vi "ConvertGoop3ToGoop4_UpdateNewVICallers.vi"(8 "error in (no error)":errorcluster, 10 "InsertAlwaysCopy":bool, 11 "ViRef":refnum<vi>) -> (0 "error out":errorcluster, 3 "ViRefOut":refnum<vi>)   [LabVIEW 2020]
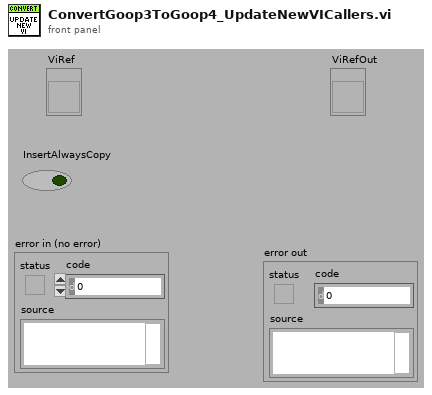
[diagram p1: front panel]
types:
  T1 = enum16{"Create or look up existing", "Look up existing"}
  T2 = enum16{"Create", "Create or look up existing", "Look up existing"}
  T3 = enum32{"invalid lock state", "Not Locked", "Locked (No Password)", "Password-protected"}
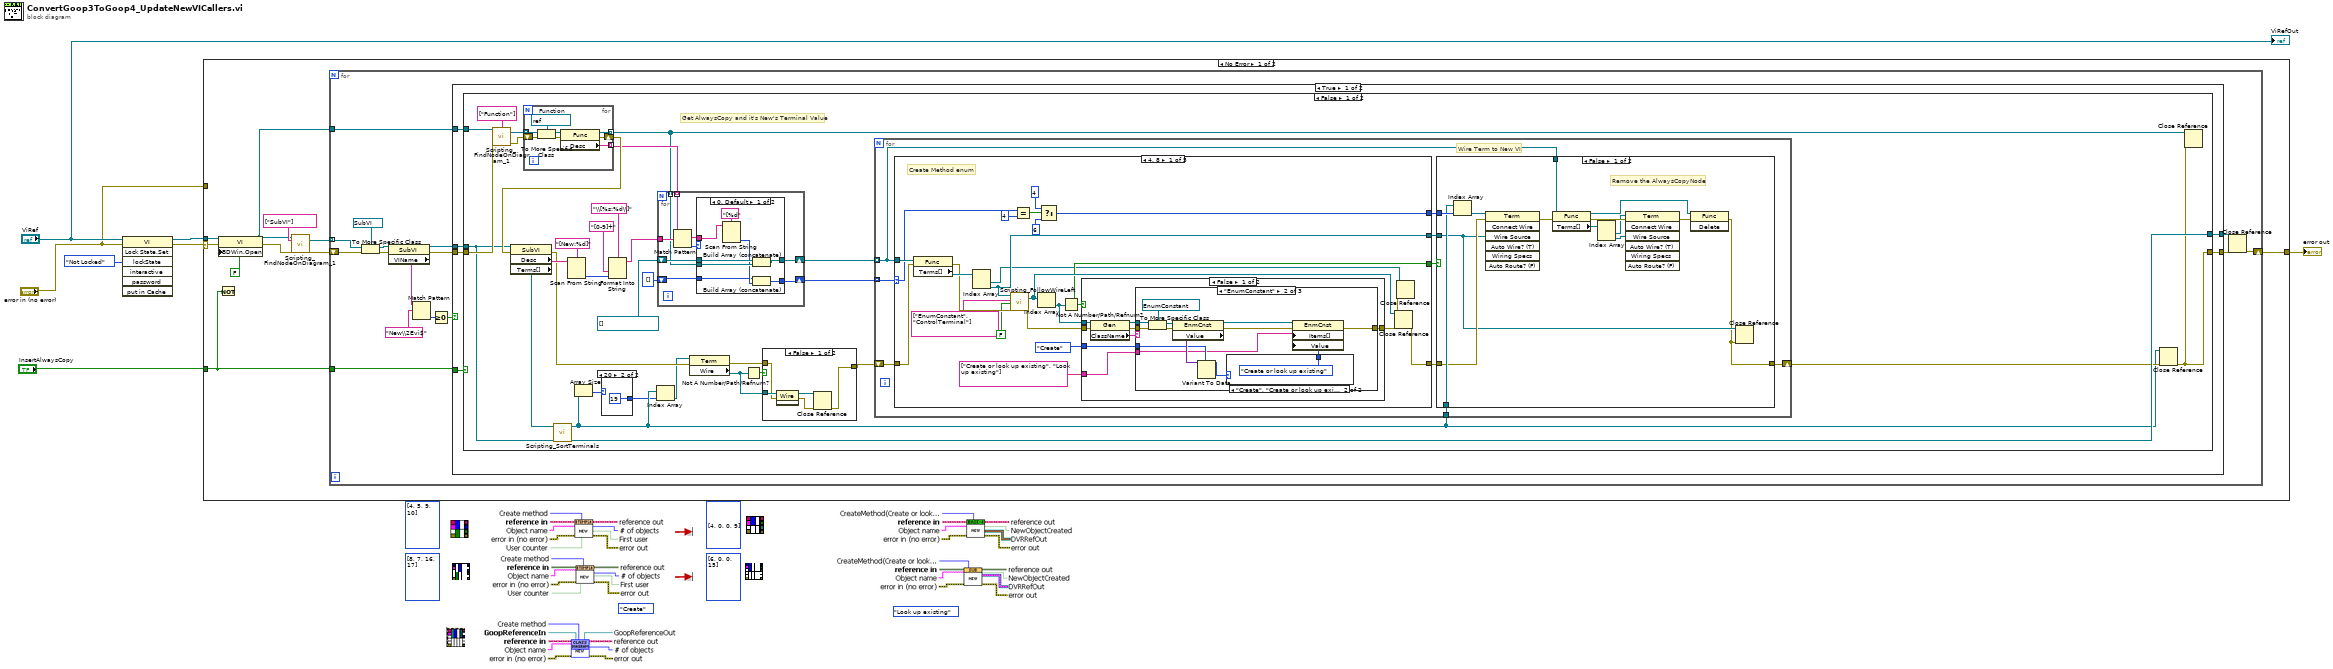
[diagram p0: block diagram]
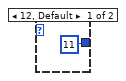
[diagram p3: hidden frame]
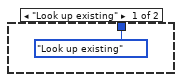
[diagram p6: hidden frame]
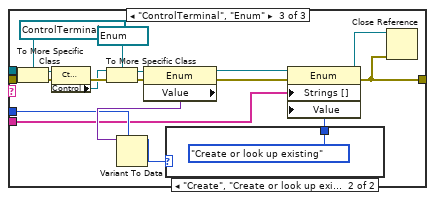
[diagram p7: hidden frame]
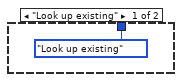
[diagram p8: hidden frame]
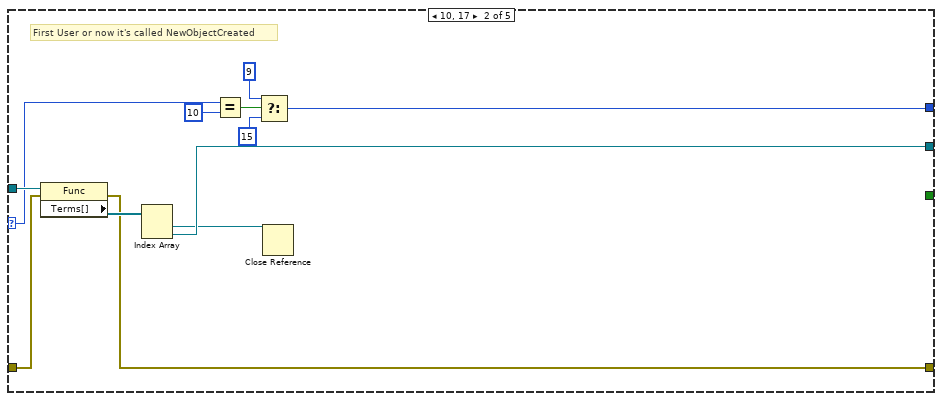
[diagram p10: hidden frame]
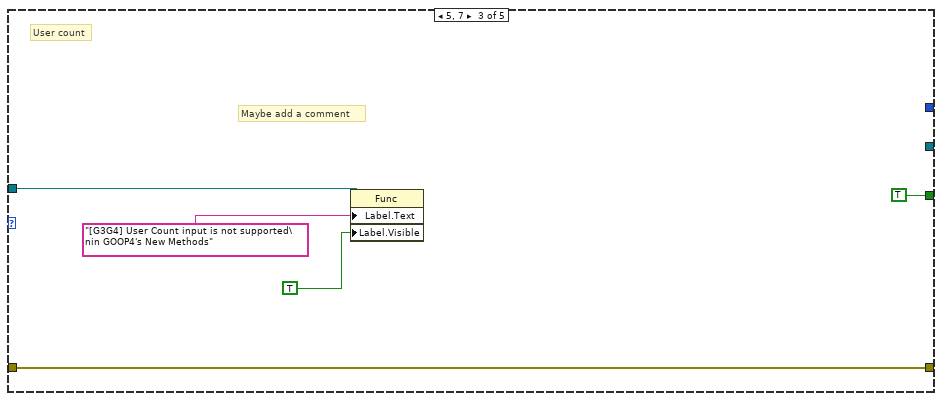
[diagram p11: hidden frame]
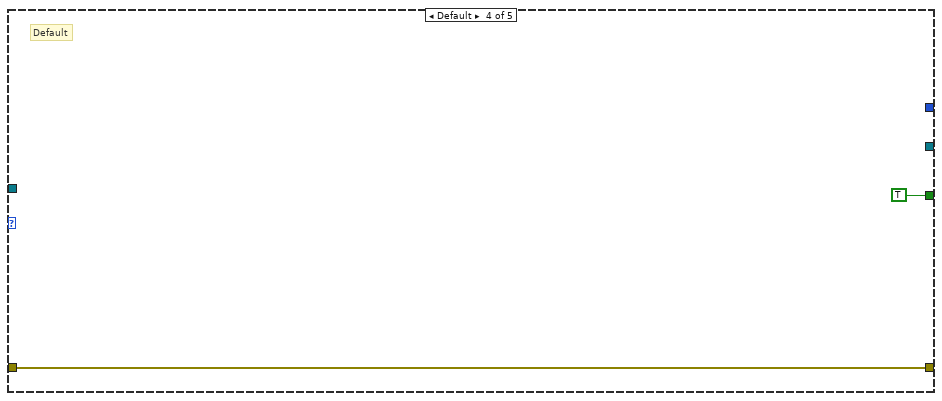
[diagram p12: hidden frame]
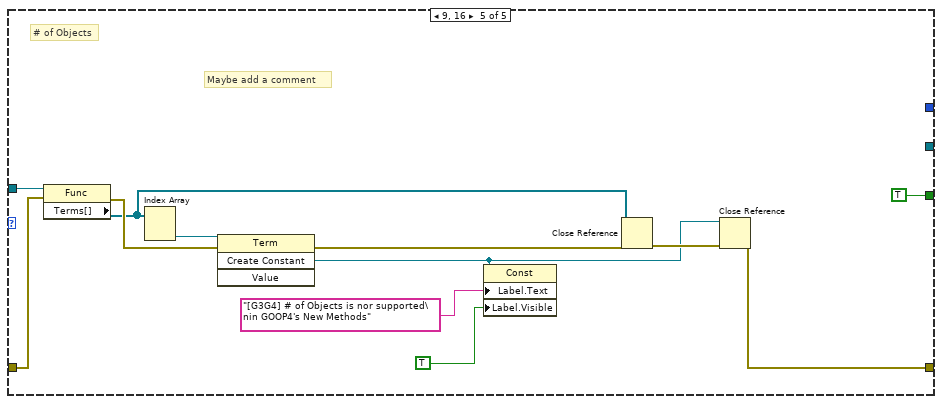
[diagram p13: hidden frame]
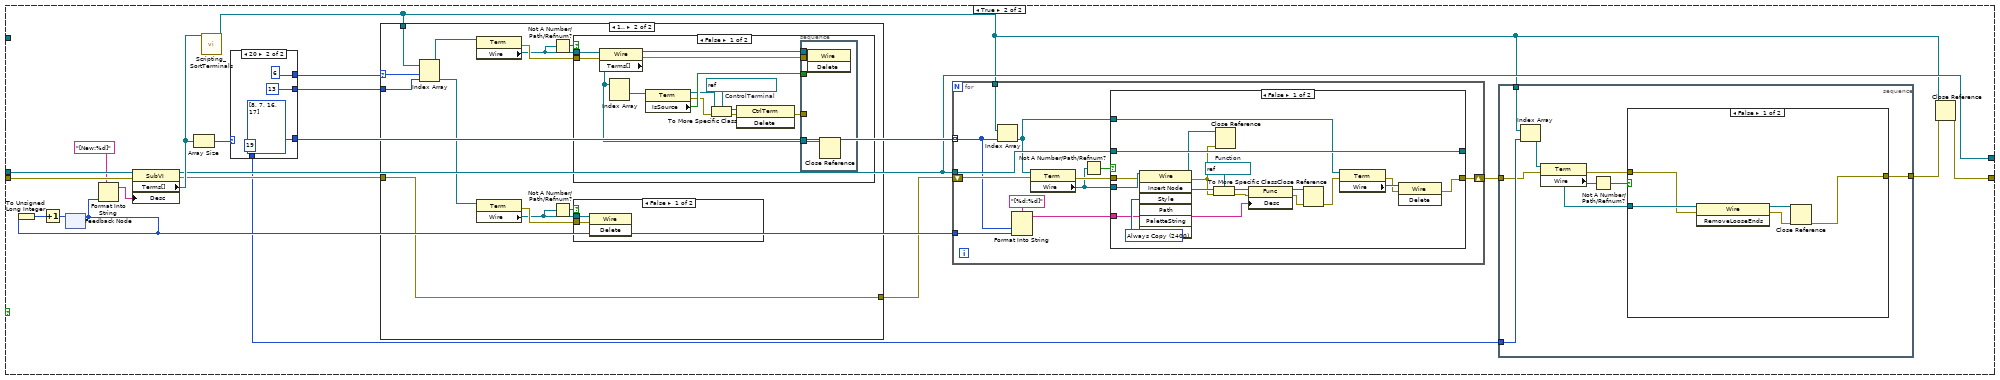
[diagram p15: hidden frame]
diagram:
  (unwired) i32[] [4, 0, 0, 9]
  (unwired) i32[] [6, 0, 0, 15]
  (unwired) T1."Look up existing" ("CreateMethod(Create or look up existing)")
  (unwired) T2."Create" ("Create method")
  (unwired) i32[] [4, 5, 9, 10]
  (unwired) i32[] [8, 7, 16, 17]
  n1 = invoke class="VI" method="Lock State.Set"(reference="ViRef", error in="error in (no error)", "lockState"=T3."Not Locked" ("Lock State")) -> (reference out=w5:refnum<vi>, error out=w2:errorcluster)  [unwired: 4 in, 5 out]
  n2 = case shown="No Error" w2 {
    selector: w2 -> [w11 _]
    tunnel: [w14 w334] -> w7
    tunnel: w5 -> [w12 _]
    tunnel: "error in (no error)" -> [_ w334]
    tunnel: "InsertAlwaysCopy" -> [w9 _]
    frame No Error {
      n3 = property class="VI"(reference=w12, error in=w11, "BDWin.Open"=FALSE ("Block Diagram Window:Open")) -> (reference out=w10:refnum<vi>, error out=w13:errorcluster)
      n4 = Not(x=w9) -> ()  [unwired: 1 out]
      n5 = call <resource>:"Scripting_FindNodeOnDiagram_1.vi"("ViRef(Ignored If Not Wired)"=w10, "NodeTypesToSearchFor"=string[] ["SubVI"], "error in (no error)"=w13) -> ("Nodes"=w16:refnum<vi>[], "error out"=w15:errorcluster)  [unwired: 15 in]
      n6 = for {
        tunnel: w16 -> [w33] mode=indexing
        shift-right: [w25] -> w14
        shift-left: w15 -> [w31]
        tunnel: w9 -> [w19]
        tunnel: w10 -> [w18]
        n7 = To More Specific Class(target class=refnum<vi> refnum ("WhileLoop"), reference=w33, error in=w31) -> (specific class reference=w30:refnum<vi>, error out=w29:errorcluster)
        n8 = property class="SubVI"(reference=w30, error in=w29) -> (reference out=w28:refnum<vi>, error out=w27:errorcluster, "VIName"=w20:string)
        n9 = Match Pattern(string=w20, regular expression="New\\2Evi$") -> (offset past match=w22:i32)  [unwired: 1 in, 3 out]
        n10 = Greater Or Equal To 0?(x=w22) -> (x >= 0?=w23:bool)
        n11 = case shown="True" w23 {
          tunnel: w28 -> [w39 w332]
          tunnel: w27 -> [w38 w333]
          tunnel: [w37 w333] -> w26
          tunnel: [w34 w332] -> w24
          tunnel: w19 -> [w36 _]
          tunnel: w18 -> [w35 _]
          frame True {
            n12 = case shown="False" w36 {
              tunnel: w39 -> [w53 w248]
              tunnel: w38 -> [w69 w245]
              tunnel: [w49 w242] -> w37
              tunnel: w35 -> [w68 _]
              tunnel: [w53 w237] -> w34
              frame False {
                # "Get AlwaysCopy and it's New's Terminal Value"
                n13 = call <resource>:"Scripting_FindNodeOnDiagram_1.vi"("ViRef(Ignored If Not Wired)"=w68, "NodeTypesToSearchFor"=string[] ["Function"], "error in (no error)"=w69) -> ("Nodes"=w67:refnum<vi>[], "error out"=w66:errorcluster)  [unwired: 15 in]
                n14 = for {
                  tunnel: w67 -> [w226] mode=indexing
                  tunnel: [w225] -> w60 mode=indexing
                  tunnel: [w224] -> w50 mode=indexing
                  shift-right: [w222] -> w65
                  shift-left: w66 -> [w223]
                  w227 = refnum<vi> refnum  # Function
                  n15 = To More Specific Class(target class=w227, reference=w226, error in=w223) -> (specific class reference=w228:refnum<vi>, error out=w221:errorcluster)
                  n16 = property class="Func"(reference=w228, error in=w221) -> (reference out=w224:refnum<vi>, error out=w222:errorcluster, "Desc"=w225:string)
                }
                n17 = property class="SubVI"(reference=w53, error in=w65) -> (error out=w45:errorcluster, "Desc"=w64:string, "Terms[]"=w52:refnum<vi>[])  [unwired: 1 out]
                n18 = call <resource>:"Scripting_SortTerminals.vi"("Terminals[]"=w52) -> ("TerminalsOut[]"=w47:refnum<vi>[])  [unwired: 8 in, 2 out]
                n19 = Scan From String(format string="[New:%d]", input string=w64) -> (output 1=w61:i32)  [unwired: 3 in, 3 out]
                n20 = Array Size(array=w47) -> (size(s)=w48:i32)
                n21 = case shown="20" w48 {
                  tunnel: [11 ("index") 19 ("index")] -> w46
                  frame 12, Default {
                  }
                  frame 20 {
                  }
                }
                n22 = Format Into String(format string="\\[%s:%d\\]", "[0-9]+" ("format string"), w61) -> (resulting string=w58:string)  [unwired: 2 in, 1 out]
                n23 = Index Array(array=w47, index=w46) -> (element=w44:refnum<vi>)
                n24 = for {
                  tunnel: w60 -> [w210] mode=indexing
                  tunnel: w58 -> [w209]
                  shift-right: [w206] -> w55
                  shift-left: refnum<vi>[] [] -> [w207]
                  tunnel: w50 -> [w205] mode=indexing
                  shift-right: [w204] -> w54
                  shift-left: i32[] [] -> [w203]
                  n25 = Match Pattern(string=w210, regular expression=w209) -> (match substring=w202:string, offset past match=w208:i32)  [unwired: 1 in, 2 out]
                  n26 = case shown="0, Default" w208 {
                    tunnel: w207 -> [w218 w220]
                    tunnel: [w217 w220] -> w206
                    tunnel: w205 -> [w216 _]
                    tunnel: w202 -> [w215 _]
                    tunnel: [w212 w219] -> w204
                    tunnel: w203 -> [w211 w219]
                    frame 0, Default {
                      n27 = Scan From String(format string="[%d", input string=w215) -> (output 1=w213:i32)  [unwired: 3 in, 3 out]
                      n28 = Build Array (concatenate)(w218, w216) -> (w217:refnum<vi>[])
                      n29 = Build Array (concatenate)(w211, w213) -> (w212:i32[])
                    }
                    frame -1 {
                    }
                  }
                }
                n30 = property class="Term"(reference=w44, error in=w45) -> (error out=w42:errorcluster, "Wire"=w40:refnum<vi>)  [unwired: 1 out]
                n31 = Not A Number/Path/Refnum?(number/path/refnum=w40) -> (NaN/Path/Refnum?=w43:bool)
                n32 = case shown="False" w43 {
                  tunnel: w40 -> [w75 _]
                  tunnel: w42 -> [w74 w76]
                  tunnel: [w71 w76] -> w41
                  frame False {
                    n33 = invoke class="Wire" method="RemoveLooseEnds"(reference=w75, error in=w74) -> (reference out=w73:refnum<vi>, error out=w72:errorcluster)  [unwired: 1 in, 1 out]
                    n34 = Close Reference(reference=w73, error in (no error)=w72) -> (error out=w71:errorcluster)
                  }
                  frame True {
                  }
                }
                n35 = for {
                  tunnel: w55 -> [w80] mode=indexing
                  tunnel: w54 -> [w87] mode=indexing
                  shift-right: [w79] -> w51
                  shift-left: w41 -> [w86]
                  tunnel: w47 -> [w83]
                  # "Wire Term to New VI"
                  n36 = case shown="4, 8" w87 {
                    selector: w87 -> [w114 w179 _ _ _]
                    tunnel: w80 -> [w124 w182 w184 _ w200]
                    tunnel: w86 -> [w123 w181 w187 w189 w193]
                    tunnel: [w109 w174 _ _ _] -> w84
                    tunnel: [w108 w172 w187 w189 w194] -> w85
                    tunnel: [w107 _ TRUE TRUE TRUE] -> w81
                    tunnel: [w106 w173 _ _ _] -> w82
                    frame 4, 8 {
                      # "Create Method enum"
                      n37 = property class="Func"(reference=w124, error in=w123) -> (error out=w121:errorcluster, "Terms[]"=w122:refnum<vi>[])  [unwired: 1 out]
                      n38 = Index Array(array=w122) -> (element #1=w103:refnum<vi>, element #2=w106:refnum<vi>)  [unwired: 2 in]
                      n39 = call <resource>:"Scripting_FollowWireLeft.vi"("Term Refnum"=w106, "NodeTypesToFind"=string[] ["EnumConstant", "ControlTerminal"], "CreateParentTerminals(False)"=FALSE, "error in"=w121) -> ("Nodes"=w115:refnum<vi>[], "error out"=w117:errorcluster)  [unwired: 12 in, 2 out]
                      n40 = Equal?(x=w114, y=4) -> (x = y?=w112:bool)
                      n41 = Index Array(array=w115) -> (element=w118:refnum<vi>)  [unwired: 1 in]
                      n42 = Select(t=4 ("y"), s=w112, f=6) -> (s? t:f=w109:i32)
                      n43 = Not A Number/Path/Refnum?(number/path/refnum=w118) -> (NaN/Path/Refnum?=w107:bool)
                      n44 = case shown="False" w107 {
                        tunnel: w118 -> [w132 _]
                        tunnel: w117 -> [w131 w170]
                        tunnel: T2."Create" ("Create method") -> [w127 _]
                        tunnel: [w126 w170] -> w104
                        tunnel: string[] ["Create or look up existing", "Look up existing"] ("Items[]") -> [w125 _]
                        frame False {
                          n45 = property class="Gen"(reference=w132, error in=w131) -> (reference out=w129:refnum<vi>, error out=w128:errorcluster, "ClassName"=w130:string)
                          n46 = case shown="\"EnumConstant\"" w130 {
                            tunnel: w129 -> [_ w146 w167]
                            tunnel: w128 -> [w133 w145 w166]
                            tunnel: w127 -> [_ w138 w162]
                            tunnel: [w133 w135 w150] -> w126
                            tunnel: w125 -> [_ w134 w158]
                            frame Default {
                            }
                            frame "EnumConstant" {
                              n47 = To More Specific Class(target class=refnum<vi> refnum ("reference"), reference=w146, error in=w145) -> (specific class reference=w143:refnum<vi>, error out=w142:errorcluster)
                              n48 = property class="EnmCnst"(reference=w143, error in=w142) -> (reference out=w141:refnum<vi>, error out=w140:errorcluster, "Value"=w139:variant)
                              n49 = Variant To Data(type=w138, Variant=w139) -> (data=w137:T2)  [unwired: 1 in, 1 out]
                              n50 = case shown="\"Create\", \"Create or look up existing\", Default" w137 {
                                tunnel: [T1."Look up existing" ("CreateMethod(Create or look up existing)") T1."Create or look up existing" ("CreateMethod(Create or look up existing)")] -> w136
                                frame "Look up existing" {
                                }
                                frame "Create", "Create or look up existing", Default {
                                }
                              }
                              n51 = property class="EnmCnst"(reference=w141, error in=w140, "Items[]"=w134, "Value"=w136) -> (error out=w135:errorcluster)  [unwired: 1 out]
                            }
                            frame "ControlTerminal", "Enum" {
                              n52 = To More Specific Class(target class=refnum<vi> refnum ("reference"), reference=w167, error in=w166) -> (specific class reference=w156:refnum<vi>, error out=w155:errorcluster)
                              n53 = property class="CtrlTerm"(reference=w156, error in=w155) -> (error out=w154:errorcluster, "Control"=w151:refnum<vi>)  [unwired: 1 out]
                              n54 = To More Specific Class(target class=refnum<vi> refnum ("reference"), reference=w151, error in=w154) -> (specific class reference=w152:refnum<vi>, error out=w153:errorcluster)
                              n55 = property class="Enum"(reference=w152, error in=w153) -> (reference out=w165:refnum<vi>, error out=w164:errorcluster, "Value"=w163:variant)
                              n56 = Variant To Data(type=w162, Variant=w163) -> (data=w161:T2)  [unwired: 1 in, 1 out]
                              n57 = case shown="\"Create\", \"Create or look up existing\", Default" w161 {
                                tunnel: [T1."Look up existing" ("CreateMethod(Create or look up existing)") T1."Create or look up existing" ("CreateMethod(Create or look up existing)")] -> w160
                                frame "Look up existing" {
                                }
                                frame "Create", "Create or look up existing", Default {
                                }
                              }
                              n58 = property class="Enum"(reference=w165, error in=w164, "Strings []"=w158, "Value"=w160) -> (reference out=w149:refnum<vi>, error out=w150:errorcluster)
                              n59 = Close Reference(reference=w149, error in (no error)=w150) -> ()  [unwired: 1 out]
                            }
                          }
                        }
                        frame True {
                        }
                      }
                      n60 = Close Reference(reference=w115, error in (no error)=w104) -> (error out=w108:errorcluster)
                      n61 = Close Reference(reference=w103, error in (no error)=w104) -> ()  [unwired: 1 out]
                    }
                    frame 10, 17 {
                      # "First User or now it's called NewObjectCreated"
                      n62 = property class="Func"(reference=w182, error in=w181) -> (error out=w172:errorcluster, "Terms[]"=w180:refnum<vi>[])  [unwired: 1 out]
                      n63 = Index Array(array=w180) -> (element #1=w171:refnum<vi>, element #2=w173:refnum<vi>)  [unwired: 2 in]
                      n64 = Equal?(x=w179, y=10) -> (x = y?=w177:bool)
                      n65 = Select(t=9 ("y"), s=w177, f=15) -> (s? t:f=w174:i32)
                      n66 = Close Reference(reference=w171) -> ()  [unwired: 1 in, 1 out]
                    }
                    frame 5, 7 {
                      # "Maybe add a comment"
                      # "User count"
                      n67 = property class="Func"(reference=w184, "Label.Text"="[G3G4] User Count input is not supported\nin GOOP4's New Methods", "Label.Visible"=TRUE) -> ()  [unwired: 1 in, 2 out]
                    }
                    frame Default {
                      # "Default"
                    }
                    frame 9, 16 {
                      # "Maybe add a comment"
                      # "# of Objects"
                      n68 = property class="Func"(reference=w200, error in=w193) -> (error out=w198:errorcluster, "Terms[]"=w196:refnum<vi>[])  [unwired: 1 out]
                      n69 = Index Array(array=w196) -> (element #2=w199:refnum<vi>)  [unwired: 2 in, 1 out]
                      n70 = invoke class="Term" method="Create Constant"(reference=w199, error in=w198) -> (error out=w197:errorcluster, "Create Constant"=w192:refnum<vi>)  [unwired: 2 in, 2 out]
                      n71 = property class="Const"(reference=w192, "Label.Text"="[G3G4] # of Objects is nor supported\nin GOOP4's New Methods", "Label.Visible"=TRUE) -> ()  [unwired: 1 in, 2 out]
                      n72 = Close Reference(reference=w196, error in (no error)=w197) -> (error out=w195:errorcluster)
                      n73 = Close Reference(reference=w192, error in (no error)=w195) -> (error out=w194:errorcluster)
                    }
                  }
                  n74 = case shown="False" w81 {
                    tunnel: w85 -> [w98 w102]
                    tunnel: w84 -> [w101 _]
                    tunnel: w83 -> [w99 _]
                    tunnel: w82 -> [w89 _]
                    tunnel: w80 -> [w91 _]
                    tunnel: [w88 w102] -> w79
                    frame False {
                      # "Remove the AlwaysCopyNode"
                      n75 = Index Array(array=w99, index=w101) -> (element=w100:refnum<vi>)
                      n76 = invoke class="Term" method="Connect Wire"(reference=w100, error in=w98, "Wire Source"=w89) -> (error out=w92:errorcluster)  [unwired: 4 in, 6 out]
                      n77 = property class="Func"(reference=w91, error in=w92) -> (reference out=w97:refnum<vi>, error out=w96:errorcluster, "Terms[]"=w90:refnum<vi>[])
                      n78 = Index Array(array=w90) -> (element #1=w95:refnum<vi>, element #2=w94:refnum<vi>)  [unwired: 2 in]
                      n79 = invoke class="Term" method="Connect Wire"(reference=w95, error in=w96, "Wire Source"=w94) -> (error out=w93:errorcluster)  [unwired: 4 in, 6 out]
                      n80 = invoke class="Func" method="Delete"(reference=w97, error in=w93) -> (error out=w88:errorcluster)  [unwired: 1 in, 2 out]
                      n81 = Close Reference(reference=w89, error in (no error)=w88) -> ()  [unwired: 1 out]
                    }
                    frame True {
                    }
                  }
                }
                n82 = Close Reference(reference=w47, error in (no error)=w51) -> (error out=w49:errorcluster)
                n83 = Close Reference(reference=w50, error in (no error)=w49) -> ()  [unwired: 1 out]
              }
              frame True {
                n84 = feedback #1() -> (w239:u32)  [unwired: 1 in]
                n85 = To Unsigned Long Integer(number=w239) -> (unsigned 32bit integer=w243:u32)
                n86 = Increment(x=w243) -> (x+1=w244:u32)
                n87 = feedback-in #1(w244) -> ()
                n88 = Format Into String(format string="[New:%d]", w239) -> (resulting string=w238:string)  [unwired: 2 in, 1 out]
                n89 = property class="SubVI"(reference=w248, error in=w245, "Desc"=w238) -> (reference out=w237:refnum<vi>, error out=w234:errorcluster, "Terms[]"=w247:refnum<vi>[])
                n90 = Array Size(array=w247) -> (size(s)=w246:i32)
                n91 = call <resource>:"Scripting_SortTerminals.vi"("Terminals[]"=w247) -> ("TerminalsOut[]"=w232:refnum<vi>[])  [unwired: 8 in, 2 out]
                n92 = case shown="20" w246 {
                  tunnel: [i32[] [4, 5, 9, 10] i32[] [8, 7, 16, 17]] -> w241
                  tunnel: [_ 6 ("index")] -> w236
                  tunnel: [_ 13 ("index")] -> w235
                  tunnel: [11 ("index") 19 ("index")] -> w230
                  frame 12, Default {
                  }
                  frame 20 {
                  }
                }
                n93 = case shown="1.." w236 {
                  selector: w236 -> [_ w274]
                  tunnel: w232 -> [_ w275]
                  tunnel: w235 -> [_ w273]
                  tunnel: w234 -> [w263 w264]
                  tunnel: [w263 w264] -> w233
                  frame 0, Default {
                  }
                  frame 1.. {
                    n94 = Index Array(array=w275, index #1=w274, index #2=w273) -> (element #1=w271:refnum<vi>, element #2=w267:refnum<vi>)
                    n95 = property class="Term"(reference=w271) -> (error out=w272:errorcluster, "Wire"=w270:refnum<vi>)  [unwired: 1 in, 1 out]
                    n96 = property class="Term"(reference=w267) -> (error out=w268:errorcluster, "Wire"=w266:refnum<vi>)  [unwired: 1 in, 1 out]
                    n97 = Not A Number/Path/Refnum?(number/path/refnum=w270) -> (NaN/Path/Refnum?=w269:bool)
                    n98 = Not A Number/Path/Refnum?(number/path/refnum=w266) -> (NaN/Path/Refnum?=w265:bool)
                    n99 = case shown="False" w269 {
                      tunnel: w272 -> [w289 _]
                      tunnel: w270 -> [w290 _]
                      frame False {
                        w285 = refnum<vi> refnum  # ControlTerminal
                        n100 = property class="Wire"(reference=w290, error in=w289) -> (reference out=w288:refnum<vi>, error out=w287:errorcluster, "Terms[]"=w281:refnum<vi>[])
                        n101 = Index Array(array=w281) -> (element #1=w286:refnum<vi>)  [unwired: 2 in, 1 out]
                        n102 = property class="Term"(reference=w286) -> (reference out=w279:refnum<vi>, error out=w278:errorcluster, "IsSource"=w280:bool)  [unwired: 1 in]
                        n103 = To More Specific Class(target class=w285, reference=w279, error in=w278) -> (specific class reference=w284:refnum<vi>, error out=w283:errorcluster)
                        n104 = invoke class="CtrlTerm" method="Delete"(reference=w284, error in=w283) -> (error out=w282:errorcluster)  [unwired: 1 in, 2 out]
                        n105 = stacked-sequence {
                          tunnel: w288 -> [w293]
                          tunnel: w287 -> [w292]
                          tunnel: w282 -> [_]
                          tunnel: w281 -> [w291]
                          tunnel: w280 -> [_]
                          frame #0 {
                            n106 = invoke class="Wire" method="Delete"(reference=w293, error in=w292) -> ()  [unwired: 1 in, 3 out]
                            n107 = Close Reference(reference=w291) -> ()  [unwired: 1 in, 1 out]
                          }
                        }
                      }
                      frame True {
                      }
                    }
                    n108 = case shown="False" w265 {
                      tunnel: w268 -> [w277 _]
                      tunnel: w266 -> [w276 _]
                      frame False {
                        n109 = invoke class="Wire" method="Delete"(reference=w276, error in=w277) -> ()  [unwired: 1 in, 3 out]
                      }
                      frame True {
                      }
                    }
                  }
                }
                n110 = for {
                  tunnel: w232 -> [w303]
                  tunnel: w237 -> [w298]
                  tunnel: w241 -> [w296] mode=indexing
                  tunnel: w239 -> [w295]
                  shift-right: [w302] -> w231
                  shift-left: w233 -> [w299]
                  n111 = Index Array(array=w303, index=w296) -> (element=w294:refnum<vi>)
                  n112 = Format Into String(format string="[%d:%d]", w296, w295) -> (resulting string=w297:string)  [unwired: 2 in, 1 out]
                  n113 = property class="Term"(reference=w294, error in=w299) -> (error out=w305:errorcluster, "Wire"=w301:refnum<vi>)  [unwired: 1 out]
                  n114 = Not A Number/Path/Refnum?(number/path/refnum=w301) -> (NaN/Path/Refnum?=w300:bool)
                  n115 = case shown="False" w300 {
                    tunnel: w305 -> [w315 w325]
                    tunnel: w297 -> [w317 _]
                    tunnel: [w306 w325] -> w302
                    tunnel: w301 -> [w319 _]
                    tunnel: w298 -> [w314 w324]
                    tunnel: [w314 w324] -> _
                    tunnel: w294 -> [w309 _]
                    frame False {
                      w320 = refnum<vi> refnum  # Function
                      w323 = 2400 items=[".NET Container"=2125, ".NET Refnum"=3441, "2D Picture"=3508, "3D Picture"=23776, "Absolute Value"=1054, "Access Rights"=1412, "ActiveX Container"=2072, "Add"=3915, "Add 1"=1050, "Add Array Elements"=1903, "Agitator"=3831, "AllSpoll"=1960, "Always Copy"=2400, "And"=1061, "And Array Elements"=1911, "Append True/False String"=1511, "Application Refnum"=3412, "Array"=21608, "Array 1"=3300, "Array Constant"=2070, "Array Interface Control"=23777, "Array Max & Min"=1907, "Array Size"=1809, "Array Subset"=2044, "Array To Cluster"=1168, "Array To Spreadsheet String"=1540, "Array of Strings to Path"=1422, "Atmospheric Tank"=3070, "Atmospheric Tank 1"=21751, "Automation Close"=8001, "Automation Open"=8000, "Automation Refnum"=3410, "Avogadro Constant (1/mol)"=23520, "Base 10 Logarithm Of e"=23512, "Bin"=3073, "Bin 1"=21755, "Bitpack to Array"=3135, "Blocking Variable Read"=23786, "Blocking Variable Write"=23789, "Bluetooth Close Connection"=9148, "Bluetooth Create Listener"=9151, "Bluetooth Discover"=9152, "Bluetooth Network Connection Refnum"=3468, "Bluetooth Open Connection"=9153, "Bluetooth Read"=9149, "Bluetooth Wait On Listener"=9147, "Bluetooth Write"=9150, "Boolean Array To Number"=1815, "Boolean To (0,1)"=1167, "Build Array"=2041, "Build Cluster Array"=2047, "Build Matrix"=8500, "Build Path"=1419, "Build Waveform"=2066, "Bundle"=2049, "Bundle By Name"=2057, "Byte Array To String"=1609, "Byte Stream File Refnum"=3408, "CAN Channel"=21966, "CAN Channel 1"=3340, "CAN Channel 2"=2124, "CAN Channel 3"=21817, "CAN Interface"=3339, "CAN Interface 1"=21815, "CAN Interface 2"=2123, "CAN Interface 3"=21964, "CAN Task"=3470, "CAN Task 1"=3471, "CAN Task 2"=21963, "CAN Task 3"=21789, "CPU Information"=24130, "Call By Reference Node"=3901, "Call Chain"=1999, "Call Library Function Node"=2062, "Call Parent Method"=2354, "Cancel Button"=21739, "Cancel Notification"=9107, "Carriage Return Constant"=23500, "Case Structure"=2001, "Cast Unit Bases"=1079, "Check Valve"=3833, "Checkbox"=3117, "Class Specifier Constant"=2094, "Classic Radio Buttons"=22003, "Clear Fixed-Point Overflow Status"=5562, "Close File"=1405, "Close File 1"=8052, "Close Reference"=8011, "Close Variable Connection"=23783, "Cluster"=3400, "Cluster 1"=21607, "Cluster Constant"=2071, "Cluster To Array"=1169, "Code Interface Node"=2050, "Coerce To Type"=2402, "Color Box"=3013, "Color Box Constant"=2120, "Color Box Thin Border"=2905, "Color Ramp"=3022, "Combo Box"=21604, "Combo Box 1"=3304, "Combo Box Constant"=2088, "Complex Conjugate"=1048, "Complex To Polar"=1045, "Complex To Re/Im"=1044, "Compound Arithmetic"=2200, "Compressor"=3832, "Concatenate Strings"=2040, "Conditional Disable Structure"=2064, "Constructor Node"=3904, "Control & Simulation Loop"=2099, "Control Help Window"=1353, "Control Online Help"=1355, "Control Refnum"=3419, "Convert Unit"=2059, "Conveyer"=3827, "Copy"=1416, "Copy 1"=8053, "Cosecant"=1204, "Cosine"=1201, "Cotangent"=1205, "Create Folder"=8055, "Create User Event"=2073, "Current Processor ID"=24131, "Current VI's Menubar"=9000, "Current VI's Path"=1426, "DAQmx Analog Trigger Source"=3336, "DAQmx Analog Trigger Source 1"=2119, "DAQmx Analog Trigger Source 2"=21951, "DAQmx Analog Trigger Source 3"=21774, "DAQmx Device Name"=21773, "DAQmx Device Name 1"=21950, "DAQmx Device Name 2"=2093, "DAQmx Device Name 3"=3318, "DAQmx Global Channel"=3443, "DAQmx Global Channel 1"=21770, "DAQmx Global Channel 2"=21957, "DAQmx Global Channel 3"=3430, "DAQmx Physical Channel"=3335, "DAQmx Physical Channel 1"=21954, "DAQmx Physical Channel 2"=2118, "DAQmx Physical Channel 3"=21777, "DAQmx Scale Name"=21952, "DAQmx Scale Name 1"=21775, "DAQmx Scale Name 2"=3317, "DAQmx Scale Name 3"=2116, "DAQmx Switch"=21953, "DAQmx Switch 1"=3337, "DAQmx Switch 2"=2121, "DAQmx Switch 3"=21776, "DAQmx Task Name"=3442, "DAQmx Task Name 1"=3434, "DAQmx Task Name 2"=21959, "DAQmx Task Name 3"=21778, "DAQmx Terminal"=21955, "DAQmx Terminal 1"=2117, "DAQmx Terminal 2"=21781, "DAQmx Terminal 3"=3319, "Data Cache Size"=24132, "Data Log File Refnum"=3402, "DataSocket Close"=1085, "DataSocket Open"=1084, "DataSocket Read"=1086, "DataSocket Refnum"=3417, "DataSocket Write"=1087, "Date/Time To Seconds"=1308, "Decimal Digit?"=1119, "Decimal String To Number"=1184, "Decimate 1D Array"=2046, "DecomposeArray"=2412, "DecomposeLockDataValRef"=2406, "DecomposeVariant"=2404, "Decrement"=1058, "Default Directory"=1427, "Delete"=8056, "Delete 1"=1417, "Delete Data Value Reference"=2409, "Delete From Array"=3912, "Delete Menu Items"=9004, "Delete Variant Attribute"=8206, "Delete Waveform Attribute"=8209, "Deny Access"=8057, "Dequeue Element"=9113, "Destroy User Event"=2075, "DevClear"=1961, "DevClearList"=1962, "Device Control/Status"=1433, "Device Refnum"=3405, "Diagram Disable Structure"=2054, "Dial"=3050, "Dial 1"=21732, "Digital Data"=3210, "Digital Data 1"=21216, "Digital Waveform Graph"=21718, "Digital Waveform Graph 1"=3511, "Direct Variable Read"=23785, "Direct Variable Write"=23788, "Divide"=1053, "Divide 1"=3918, "Dlg CheckBox"=21924, "Dlg Horiz Scrollbar"=21905, "Dlg Numeric"=2100, "Dlg Numeric 2"=3006, "Dlg String"=2110, "Dlg Vert Scrollbar"=21906, "Down Arrow"=3824, "Down Bow Valve"=3707, "Down Bow Valve 1"=21767, "Down Bow Valve 2"=3807, "Down Rect Valve"=21766, "Down Rect Valve 1"=3706, "Down Rect Valve 2"=3806, "Down Tee"=3818, "Down Tee 1"=3718, "EOF"=1410, "Elementary Charge (C)"=23517, "Empty Array?"=23063, "Empty Path Constant"=23523, "Empty String Constant"=23503, "Empty String/Path?"=1112, "Enable Menu Tracking"=9002, "EnableLocal"=1963, "EnableRemote"=1964, "End of Line Constant"=23525, "Enqueue Element"=9111, "Enqueue Element At Opposite End"=9129, "Enum"=3023, "Enum 1"=21605, "Enum Constant"=2090, "Equal To 0?"=1113, "Equal?"=1102, "Error Ring Constant"=2039, "Event Callback Refnum"=3435, "Event Data Node"=2102, "Event Structure"=2052, "Exchanger"=3828, "Exclusive Or"=1063, "Exponential"=1211, "Exponential (Arg) -1"=1222, "Expression Node"=2201, "FIFO Refnum"=3474, "False Constant"=2006, "Feedback Node, Feedback Node 1"=2353, "FieldPoint IO Point"=21784, "FieldPoint IO Point 1"=3440, "FieldPoint IO Point 2"=3439, "File Dialog"=8058, "File Dialog 1"=8081, "File Path Control"=21730, "File Path Control 1"=3203, "File Path Indicator"=21731, "File Path Indicator 1"=3204, "File/Directory Info"=1413, "File/Directory Info 1"=8082, "FindLstn"=1965, "FindRQS"=1966, "First Call?"=1083, "Fixed-Point Overflow?"=5565, "Fixed-Point to Integer Cast"=5566, "Flat Box"=3602, "Flat Circle"=3605, "Flat Down Triangle"=3623, "Flat Frame"=3608, "Flat Left Triangle"=3620, "Flat Right Triangle"=3621, "Flat Round Button"=3102, "Flat Rounded Box"=3611, "Flat Sequence Structure"=2069, "Flat Square Button"=3103, "Flat Up Triangle"=3622, "Flatten To String"=1164, "Flatten To XML"=8400, "Flattened String To Variant"=8202, "Floating Point Equal?"=23064, "Flush File"=8059, "Flush File 1"=1406, "Flush Queue"=9114, "For Loop"=2002, "Fork"=2194, "Format Date/Time String"=8100, "Format Into File"=2083, "Format Into String"=2081, "Format Value"=1512, "Formula Node"=2004, "Fract/Exp String To Number"=1187, "Framed Color Box"=21019, "Framed Color Box 1"=3008, "Free Label"=2321, "Furnace"=3829, "GPIB Clear"=1954, "GPIB Initialization"=1957, "GPIB Misc"=1956, "GPIB Read"=1951, "GPIB Serial Poll"=1955, "GPIB Status"=1959, "GPIB Trigger"=1953, "GPIB Wait"=1958, "GPIB Write"=1950, "Gauge"=21009, "Gauge 1"=3040, "Generate Front Panel Activity"=1329, "Generate Occurrence"=1700, "Generate User Event"=2074, "Generate User-Defined Trace Event"=2250, "Get Datalog Position"=8061, "Get Date/Time In Seconds"=1303, "Get Date/Time String"=1600, "Get Drag Drop Data"=9154, "Get File Position"=8062, "Get File Size"=8063, "Get Fixed-Point Components"=11163, "Get Help Window Status"=1354, "Get Matrix Diagonal"=8501, "Get Matrix Elements"=8502, "Get Menu Item Info"=9005, "Get Menu Selection"=9001, "Get Menu Short Cut Info"=9007, "Get Notifier Status"=9103, "Get Number of Records"=8064, "Get Permissions"=8065, "Get Queue Status"=9110, "Get Submatrix"=8503, "Get Type and Creator"=8066, "Get Variant Attribute"=8205, "Get Volume Info"=8067, "Get Waveform Attribute"=8208, "Get Waveform Components"=2067, "Global Variable"=2060, "Gravitational Constant (N m2/kg2)"=23519, "Greater Or Equal To 0?"=1114, "Greater Or Equal?"=1103, "Greater Than 0?"=1117, "Greater?"=1110, "Handle Peek"=1604, "Handle Poke"=1605, "Hex Digit?"=1123, "Hexadecimal String To Number"=1185, "Hopper"=21754, "Hopper 1"=3072, "Horiz Line"=3821, "Horiz Pipe"=3710, "Horiz Pipe 1"=3810, "Horizontal Button Box"=3636, "Horizontal Fill Slide"=3012, "Horizontal Fill Slide 1"=21100, "Horizontal Graduated Bar"=21106, "Horizontal Pointer Slide"=21101, "Horizontal Pointer Slide 1"=3011, "Horizontal Progress Bar"=21102, "Horizontal Scrollbar"=21110, "Horizontal Slide"=3010, "Horizontal Slide Switch"=3114, "Horizontal Smooth Box"=3633, "Horizontal Splitter Bar"=21861, "Horizontal Splitter Bar (Classic)"=21863, "Horizontal Splitter Bar (System)"=21865, "Horizontal Switch"=3108, "Horizontal Tank"=3071, "Horizontal Toggle Switch"=3110, "Horizontal Toggle Switch 1"=21700, "Hyperbolic Cosecant"=23053, "Hyperbolic Cosine"=1215, "Hyperbolic Cotangent"=23055, "Hyperbolic Secant"=23054, "Hyperbolic Sine"=1214, "Hyperbolic Tangent"=1216, "IMAQ Session"=3415, "IP To String"=1710, "IVI Delete Session"=8103, "IVI Logical Name"=3420, "IVI Logical Name 1"=3414, "IVI Logical Name 2"=21736, "IVI New Session"=8102, "Implies"=1080, "In Place Element Structure"=2360, "In Range and Coerce"=1127, "Include Fixed-Point Overflow Status"=5564, "Increment"=1057, "Index & Bundle Cluster Array"=2056, "Index Array"=2042, "Index String Array"=1531, "Initialize Array"=2053, "Inline C Node"=2104, "Insert Into Array"=3911, "Insert Menu Items"=9003, "Integer to Fixed-Point Cast"=5567, "Intensity Chart"=21719, "Intensity Chart 1"=3509, "Intensity Graph"=21720, "Intensity Graph 1"=3510, "Interleave 1D Arrays"=2045, "Interpolate 1D Array"=1905, "Inverse Cosecant"=23050, "Inverse Cosine"=1207, "Inverse Cotangent"=23052, "Inverse Hyperbolic Cosecant"=23056, "Inverse Hyperbolic Cosine"=1218, "Inverse Hyperbolic Cotangent"=23058, "Inverse Hyperbolic Secant"=23057, "Inverse Hyperbolic Sine"=1217, "Inverse Hyperbolic Tangent"=1219, "Inverse Secant"=23051, "Inverse Sine"=1206, "Inverse Tangent"=1208, "Inverse Tangent (2 Input)"=1228, "Invoke Node"=3900, "IrDA Close Connection"=9144, "IrDA Create Listener"=9140, "IrDA Discover"=9141, "IrDA Network Connection Refnum"=3450, "IrDA Open Connection"=9142, "IrDA Read"=9145, "IrDA Wait On Listener"=9143, "IrDA Write"=9146, "Join"=2195, "Join Numbers"=1171, "Junction"=2197, "Knob"=21000, "Knob 1"=3005, "LED Button"=3116, "LabVIEW Object"=3457, "Label"=21960, "Labeled Oblong Button"=3125, "Labeled Rectangular Button"=3124, "Labeled Round Button"=3122, "Labeled Square Button"=3123, "Leak Variant Value Reference"=2410, "Left Arrow"=3826, "Left Bow Valve"=3701, "Left Bow Valve 1"=3801, "Left Bow Valve 2"=21761, "Left Down Elbow"=3711, "Left Down Elbow 1"=3811, "Left Pump"=3713, "Left Pump 1"=3813, "Left Rect Valve"=3700, "Left Rect Valve 1"=21760, "Left Rect Valve 2"=3800, "Left Tee"=3709, "Left Tee 1"=3809, "Left Up Elbow"=3808, "Left Up Elbow 1"=3708, "Less Or Equal To 0?"=1115, "Less Or Equal?"=1104, "Less Than 0?"=1118, "Less?"=1111, "Lexical Class"=1126, "Line Feed Constant"=23501, "List Directory"=1418, "List Folder"=8083, "Listbox"=21792, "Listbox 1"=21806, "Listbox Symbol Ring Constant"=2038, "Local Variable"=2061, "Lock Range"=1411, "Logarithm Base 10"=1210, "Logarithm Base 2"=1225, "Logarithm Base X"=1224, "Logical Shift"=1081, "Lossy Enqueue Element"=9130, "Lowered Rounded Box"=3638, "MATLAB script"=9020, "Machine Epsilon"=23528, "MakeAddr"=1967, "Mantissa & Exponent"=1150, "Match First String"=1532, "Match Pattern"=1535, "Match True/False String"=1533, "MathScript Call By Reference Node"=3906, "MathScript Node"=2357, "Matrix Size"=8507, "Max & Min"=1108, "Menu Refnum"=3413, "Menu Ring"=3018, "Menu Ring 1"=21600, "Menu-Popup Ring"=3017, "Merge Signals"=2350, "Meter"=21008, "Meter 1"=3030, "Mixed Signal Graph"=21721, "Molar Gas Constant (J/(mol K))"=23522, "Motion Resource"=21787, "Motion Resource 1"=3448, "Motion Resource 2"=3449, "Motor"=3720, "Motor 1"=3820, "Move"=1415, "Move 1"=8068, "Multi-Segment Pipe"=23780, "Multicolumn Listbox"=21799, "Multicolumn Listbox 1"=21791, "Multiple Selection Listbox"=3208, "Multiply"=1052, "Multiply 1"=3917, "Multiply Array Elements"=1904, "Multirate Structure"=2199, "Natural Logarithm"=1209, "Natural Logarithm (Arg +1)"=1221, "Natural Logarithm Base"=23510, "Natural Logarithm Of 10"=23513, "Natural Logarithm Of 2"=23514, "Natural Logarithm Of Pi"=23508, "Negate"=1069, "Negative Infinity"=23509, "New Data Value Reference"=2408, "New Directory"=1402, "New File"=1404, "New VI"=8014, "New VI Object"=8015, "Not"=1064, "Not A Number/Path/Refnum?"=1128, "Not A Path Constant"=23524, "Not And"=1071, "Not Equal To 0?"=1116, "Not Equal?"=1105, "Not Exclusive Or"=1073, "Not Or"=1072, "Not a Refnum Constant"=23526, "Not a Shared Variable"=23527, "Notifier Refnum"=3423, "Number To Boolean Array"=1814, "Number To Decimal String"=1180, "Number To Engineering String"=1183, "Number To Exponential String"=1505, "Number To Fractional String"=1506, "Number To Hexadecimal String"=1181, "Number To Octal String"=1182, "Number of Cache Levels"=24133, "Numeric Constant"=2005, "Numeric Control"=3000, "Numeric Control 1"=21003, "Numeric Indicator"=3001, "Numeric Indicator 1"=21004, "OK Button"=21738, "OLE Variant"=3150, "Obtain Notifier"=9101, "Obtain Queue"=9108, "Occurrence Refnum"=3406, "Octal Digit?"=1129, "Octal String To Number"=1186, "Old VISA Open"=1921, "One Button Dialog"=1340, "Open Application Reference"=8012, "Open Device"=1430, "Open File"=1403, "Open Tank"=21752, "Open Tank 1"=3074, "Open VI Object Reference"=8013, "Open VI Reference"=8010, "Open Variable Connection"=23779, "Open Variable Connection in Background"=23791, "Open and Verify Variable Connection"=23790, "Open/Create/Replace Datalog"=8054, "Open/Create/Replace File"=8050, "Or"=1062, "Or Array Elements"=1910, "PPoll"=1969, "PPollConfig"=1970, "PPollUnconfig"=1971, "Package Matrix"=23001, "PassControl"=1968, "Path Constant"=2009, "Path To String"=1077, "Path Type"=1421, "Path to Array of Strings"=1423, "Pi"=23504, "Pi Divided By 2"=23506, "Pi Multiplied By 2"=23505, "Pick Line"=1510, "Pict Ring"=21602, "Pict Ring 1"=3015, "PixMap"=3505, "PixMap (Do not touch it!!)"=3507, "Planck's Constant (J/Hz)"=23516, "Platform Flat Square Button"=3134, "Plug-In Control"=21820, "Polar To Complex"=1047, "Polar To Re/Im"=23061, "Positive Infinity"=23515, "Power Of 10"=1212, "Power Of 2"=1223, "Power Of X"=1213, "Preserve Run-Time Class"=8018, "Pressure Tank"=3075, "Pressure Tank 1"=21753, "Preview Queue Element"=9112, "Printable?"=1124, "Property Node"=1920, "Pulldown Menu Ring"=3061, "Push Button"=21001, "Queue Refnum"=3424, "Quit LabVIEW"=1352, "Quotient & Remainder"=1056, "RT FIFO Create"=24000, "RT FIFO Delete"=24003, "RT FIFO Read"=24001, "RT FIFO Write"=24002, "Radio Buttons"=22001, "Raised Box"=3600, "Raised Box 1"=3637, "Raised Circle"=3603, "Raised Down Triangle"=3615, "Raised Frame"=3606, "Raised Left Triangle"=3612, "Raised Right Triangle"=3613, "Raised Rounded Box"=3609, "Raised Up Triangle"=3614, "Random Number (0-1)"=1070, "RcvRespMsg"=1972, "Re/Im To Complex"=1046, "Re/Im To Polar"=23060, "Read Datalog"=8069, "Read Device"=1432, "Read File"=1407, "Read Variable"=23781, "Read from Binary File"=8051, "Read from Text File"=8070, "ReadStatus"=1973, "Receive"=1974, "ReceiveSetup"=1975, "Recessed Box"=3601, "Recessed Circle"=3604, "Recessed Down Triangle"=3619, "Recessed Frame"=3607, "Recessed Left Triangle"=3616, "Recessed Menu Ring"=3019, "Recessed Right Triangle"=3617, "Recessed Rounded Box"=3610, "Recessed Up Triangle"=3618, "Reciprocal"=1059, "Reciprocal Of Pi"=23507, "Reciprocal Of e"=23511, "RecomposeArray"=2403, "RecomposeUnlockDataValRef"=2407, "RecomposeVariant"=2405, "Rectangular Stop Button"=3128, "Refnum to Path"=1424, "Refnum to Session"=2306, "Region"=2196, "Register Event Callback"=2078, "Register For Events"=2065, "Register Session"=2319, "Release Notifier"=9102, "Release Queue"=9109, "Remove Fixed-Point Overflow Status"=5563, "Replace Array Subset"=3910, "Replace Substring"=3913, "Request Deallocation"=1610, "ResetSys"=1976, "Reshape Array"=2055, "Resize Matrix"=8508, "Reverse 1D Array"=1900, "Reverse String"=1537, "Right Arrow"=3825, "Right Bow Valve"=21765, "Right Bow Valve 1"=3705, "Right Bow Valve 2"=3805, "Right Down Elbow"=3817, "Right Down Elbow 1"=3717, "Right Pump"=3719, "Right Pump 1"=3819, "Right Rect Valve"=3804, "Right Rect Valve 1"=3704, "Right Rect Valve 2"=21764, "Right Tee"=3715, "Right Tee 1"=3815, "Right Up Elbow"=3814, "Right Up Elbow 1"=3714, "Ring Constant"=2008, "Rocker"=21002, "Rotary Feeder"=3830, "Rotate"=1082, "Rotate 1D Array"=1906, "Rotate Left With Carry"=1606, "Rotate Right With Carry"=1607, "Rotate String"=1536, "Round Button"=3100, "Round LED"=3120, "Round LED 1"=21012, "Round Light"=3104, "Round Push Button"=3112, "Round Push Button 2"=3118, "Round Radio Button"=3106, "Round Stop Button"=3127, "Round To Nearest"=1055, "Round Toward +Infinity"=1076, "Round Toward -Infinity"=1075, "Rydberg Constant (1/m)"=23521, "Scale By Power Of 2"=1074, "Scan From File"=2082, "Scan From String"=2080, "Scan String For Tokens"=8101, "Scan Value"=1534, "Scanned Variable Read"=23784, "Scanned Variable Write"=23787, "Search 1D Array"=1901, "Search and Replace String"=3914, "Search/Split String"=1538, "Secant"=1203, "Seconds To Date/Time"=1309, "Seek"=1409, "Select"=1516, "Send"=1977, "Send Notification"=9104, "SendCmds"=1978, "SendDataBytes"=1979, "SendIFC"=1980, "SendLLO"=1982, "SendList"=1981, "SendSetup"=1983, "Session to Refnum"=2307, "Set Datalog Position"=8072, "Set File Position"=8073, "Set File Size"=8074, "Set Matrix Diagonal"=8504, "Set Matrix Elements"=8505, "Set Menu Item Info"=9006, "Set Number of Records"=8075, "Set Occurrence"=1702, "Set Permissions"=8076, "Set Submatrix"=8506, "Set Type and Creator"=8077, "Set Variant Attribute"=8204, "Set Waveform Attribute"=8207, "SetRWLS"=1984, "SetTimeOut"=1985, "Shared Variable"=23778, "Shared Variable Constant"=3473, "Shared Variable Control"=3472, "Shared Variable Control 1"=21814, "Shared Variable to String"=1831, "Sign"=1049, "Simple Horizontal Slide"=3003, "Simple Numeric"=3029, "Simple Numeric 1"=2900, "Simple String"=2115, "Simple Vertical Slide"=3002, "Sinc"=1227, "Sine"=1200, "Sine & Cosine"=1220, "Size Handle"=1603, "Slide Switch"=21011, "Sort 1D Array"=1120, "Sort Array of String, Sort Array of String 1"=23065, "Speed Of Light In Vacuum (m/sec)"=23518, "Split 1D Array"=1908, "Split Button"=21020, "Split Number"=1170, "Split Signals"=2351, "Spreadsheet String To Array"=1539, "Square"=23059, "Square Button"=3101, "Square LED"=3121, "Square LED 1"=21013, "Square Light"=3105, "Square Push Button"=3113, "Square Push Button 2"=3119, "Square Radio Button"=3107, "Square Root"=1060, "Stacked Sequence Structure"=2000, "State"=2198, "State Diagram"=2051, "Static VI Reference"=2084, "Stop"=1350, "Stop Button"=21230, "String Constant"=2007, "String Control"=3200, "String Control 1"=21701, "String Indicator"=3201, "String Indicator 1"=21702, "String Length"=1502, "String Subset"=1503, "String To Byte Array"=1608, "String To IP"=1711, "String To Path"=1078, "String to Shared Variable"=1830, "Strip Path"=1420, "SubPanel"=21810, "SubPanel (Classic)"=21811, "SubPanel (System)"=21823, "Subtract"=1051, "Subtract 1"=3916, "Swap Bytes"=1162, "Swap Values"=2401, "Swap Vector Element"=1912, "Swap Words"=1163, "System Button"=3130, "System Cancel Button"=3131, "System Checkbox"=3132, "System Chiseled Line"=3632, "System Colored Rectangle"=3625, "System Combo Box"=21917, "System Enum"=3062, "System Horizontal Pointer Slide"=21902, "System Horizontal Progress Bar"=21910, "System Horizontal Slide"=21904, "System Label"=21961, "System Listbox"=21805, "System Mixed Checkbox"=21333, "System Multicolumn Listbox"=21798, "System Numeric"=21919, "System Path Control"=21922, "System Pict Ring"=21925, "System Radio Button"=3133, "System Radio Buttons"=22002, "System Recessed Frame"=3624, "System Ring"=3060, "System Spin Control"=21900, "System String"=21920, "System Tab Control"=3331, "System Table"=21797, "System Time Stamp"=21967, "System Tree"=21794, "System Vertical Pointer Slide"=21901, "System Vertical Progress Bar"=21909, "System Vertical Slide"=21903, "TCP Close Connection"=1713, "TCP Create Listener"=1717, "TCP Flattened Read"=1718, "TCP Flattened Write"=1719, "TCP Flex Read"=1720, "TCP Flex Write"=1721, "TCP Network Connection Refnum"=3407, "TCP Open Connection"=1715, "TCP Read"=1716, "TCP Wait On Listener"=1712, "TCP Write"=1714, "TDMS Close"=24113, "TDMS Defragment"=24119, "TDMS File"=3477, "TDMS Flush"=24117, "TDMS Get Properties"=24115, "TDMS List Contents"=24116, "TDMS Open"=24112, "TDMS Read"=24111, "TDMS Refnum To File ID"=24120, "TDMS Set Properties"=24114, "TDMS Write"=24110, "TDMS Write IP"=24118, "Tab Constant"=23502, "Tab Control"=3330, "Tab Control 1"=3332, "Table"=21796, "Table 1"=21790, "Tag Attribute Ring"=2063, "Tangent"=1202, "Tank"=21006, "Tank 1"=3020, "Temporary Directory"=1435, "TestSRQ"=1986, "TestSys"=1987, "Text & Pict Ring"=21603, "Text & Pict Ring 1"=3016, "Text Button"=21015, "Text Ring"=21601, "Text Ring 1"=3014, "Text to UTF-8"=23066, "Thermometer"=21007, "Thermometer 1"=3021, "Thick Chiseled Line"=3630, "Thick Line"=3629, "Thick Line with Arrow"=3631, "Thick Lowered Box"=3635, "Thin Chiseled Line"=3627, "Thin Line"=3626, "Thin Line with Arrow"=3628, "Threshold 1D Array"=1909, "Tick Count (ms)"=1300, "Time Stamp Constant"=2068, "Time Stamp Control"=21913, "Time Stamp Control 1"=5555, "Time Stamp Indicator"=21914, "Time Stamp Indicator 1"=5556, "Timed Loop"=5570, "Timed Sequence"=5573, "To Byte Integer"=1140, "To Double Precision Complex"=1152, "To Double Precision Float"=1147, "To Extended Precision Complex"=1154, "To Extended Precision Float"=1149, "To Fixed-Point"=5561, "To Long Integer"=1142, "To Lower Case"=1189, "To More Generic Class"=8017, "To More Specific Class"=8016, "To OLE Variant"=8002, "To Probe String"=2413, "To Quad Integer"=1155, "To Single Precision Complex"=1151, "To Single Precision Float"=1146, "To Time Stamp"=5560, "To Unsigned Byte Integer"=1143, "To Unsigned Long Integer"=1145, "To Unsigned Quad Integer"=1156, "To Unsigned Word Integer"=1144, "To Upper Case"=1188, "To Variant"=8201, "To Word Integer"=1141, "Traditional DAQ Channel"=21733, "Traditional DAQ Channel 1"=2085, "Traditional DAQ Channel 2"=3320, "Transpose 1D Array"=23068, "Transpose 2D Array"=1902, "Transpose Matrix"=8509, "Tree"=21819, "Tree 1"=21793, "Trigger"=1988, "TriggerList"=1989, "Two Button Dialog"=1341, "Type Cast"=1166, "Type and Creator"=1434, "UDP Close"=1726, "UDP Multicast Open"=1727, "UDP Network Connection Refnum"=3418, "UDP Open"=1723, "UDP Read"=1724, "UDP Write"=1725, "UTF-8 to Text"=23067, "Unbitpack from Array"=3136, "Unbundle"=2048, "Unbundle By Name"=2058, "Unflatten From String"=1165, "Unflatten From XML"=8401, "Unleak Variant Value Reference"=2411, "Unpackage Matrix"=23000, "Unregister For Events"=2076, "Unregister Session"=2320, "Up Arrow"=3823, "Up Bow Valve"=3703, "Up Bow Valve 1"=3803, "Up Bow Valve 2"=21763, "Up Rect Valve"=3702, "Up Rect Valve 1"=21762, "Up Rect Valve 2"=3802, "Up Tee"=3712, "Up Tee 1"=3812, "User Defined Refnum"=3428, "User Defined Refnum Tag"=21745, "User Defined Refnum Tag 1"=3429, "User Defined Refnum Tag Constant"=3426, "User Defined Refnum Tag Flatten"=21747, "User Defined Refnum Tag Flatten 1"=3454, "User Defined Tag"=21749, "User Defined Tag 1"=3329, "User Defined Tag Constant"=2114, "User Item"=3506, "VI Library"=1425, "VI Refnum"=3422, "VI Server Reference"=2091, "VISA Assert Interrupt Signal"=2309, "VISA Assert Trigger"=1929, "VISA Assert Utility Signal"=2310, "VISA Clear"=1927, "VISA Close"=1922, "VISA Disable Event"=1940, "VISA Discard Events"=1941, "VISA Enable Event"=1942, "VISA Find Resource"=1923, "VISA Flush I/O Buffer"=2302, "VISA GPIB Command"=2315, "VISA GPIB Control ATN"=2316, "VISA GPIB Control REN"=2304, "VISA GPIB Pass Control"=2317, "VISA GPIB Send IFC"=2318, "VISA In 16"=1930, "VISA In 32"=1944, "VISA In 64"=2140, "VISA In 8"=1936, "VISA Lock"=1993, "VISA Map Address"=1932, "VISA Map Trigger"=2311, "VISA Memory Allocation"=1997, "VISA Memory Allocation Ex"=2146, "VISA Memory Free"=1998, "VISA Move"=2303, "VISA Move In 16"=1948, "VISA Move In 32"=1991, "VISA Move In 64"=2144, "VISA Move In 8"=1946, "VISA Move Out 16"=1949, "VISA Move Out 32"=1992, "VISA Move Out 64"=2145, "VISA Move Out 8"=1947, "VISA Open"=2308, "VISA Out 16"=1931, "VISA Out 32"=1945, "VISA Out 64"=2141, "VISA Out 8"=1937, "VISA Peek 16"=1934, "VISA Peek 32"=1995, "VISA Peek 64"=2142, "VISA Peek 8"=1938, "VISA Poke 16"=1935, "VISA Poke 32"=1996, "VISA Poke 64"=2143, "VISA Poke 8"=1939, "VISA Read"=1925, "VISA Read STB"=1928, "VISA Read To File"=2313, "VISA Refnum to Session"=2300, "VISA Resource Name"=3421, "VISA Set I/O Buffer Size"=2301, "VISA Status Description"=1924, "VISA USB Control In"=2086, "VISA USB Control Out"=2087, "VISA Unlock"=1994, "VISA Unmap Address"=1933, "VISA Unmap Trigger"=2312, "VISA VXI Cmd or Query"=2305, "VISA Wait on Event"=1943, "VISA Write"=1926, "VISA Write From File"=2314, "VISA resource name"=3409, "VISA resource name 1"=21737, "Variable Class Specifier Constant"=2106, "Variable Configuration"=3475, "Variant"=3310, "Variant To Data"=8003, "Variant To Flattened String"=8203, "Vert Line"=3822, "Vert Pipe"=3816, "Vert Pipe 1"=3716, "Vert Rocker"=21740, "Vertical Fill Slide"=21014, "Vertical Fill Slide 1"=3009, "Vertical Graduated Bar"=21107, "Vertical Pointer Slide"=21017, "Vertical Pointer Slide 1"=3007, "Vertical Progress Bar"=21104, "Vertical Scrollbar"=21111, "Vertical Slide"=3004, "Vertical Slide Switch"=21741, "Vertical Slide Switch 1"=3115, "Vertical Smooth Box"=3634, "Vertical Splitter Bar"=21860, "Vertical Splitter Bar (Classic)"=21862, "Vertical Splitter Bar (System)"=21864, "Vertical Switch"=3109, "Vertical Toggle Switch"=21005, "Vertical Toggle Switch 1"=3111, "Volume Info"=1414, "Wait (ms)"=1302, "Wait For Activity"=1722, "Wait For Front Panel Activity"=1328, "Wait Until Next ms Multiple"=1327, "Wait for GPIB RQS"=1952, "Wait on Notification"=9105, "Wait on Notification from Multiple"=9106, "Wait on Notification from Multiple with Notifier History"=9132, "Wait on Notification with Notifier History"=9131, "Wait on Occurrence"=1701, "WaitSRQ"=1990, "Waveform Chart"=21010, "Waveform Chart 1"=3501, "Waveform Chart 2"=21717, "Waveform Graph"=21703, "Waveform Graph 1"=3504, "While Loop"=2003, "While Loop 1"=2352, "White Space?"=1125, "Write Datalog"=8079, "Write Device"=1431, "Write File"=1408, "Write Variable"=23782, "Write to Binary File"=8078, "Write to Text File"=8080, "XY Graph"=21716, "XY Graph 1"=3500, "Y-th Root of X"=23062]
                      n116 = invoke class="Wire" method="Insert Node"(reference=w319, error in=w315, "Style"=w323) -> (reference out=w312:refnum<vi>, error out=w313:errorcluster, "Insert Node"=w322:refnum<vi>)  [unwired: 4 in, 4 out]
                      n117 = To More Specific Class(target class=w320, reference=w322, error in=w313) -> (specific class reference=w321:refnum<vi>, error out=w316:errorcluster)
                      n118 = Close Reference(reference=w312, error in (no error)=w313) -> ()  [unwired: 1 out]
                      n119 = property class="Func"(reference=w321, error in=w316, "Desc"=w317) -> (reference out=w318:refnum<vi>, error out=w311:errorcluster)
                      n120 = Close Reference(reference=w318, error in (no error)=w311) -> (error out=w310:errorcluster)
                      n121 = property class="Term"(reference=w309, error in=w310) -> (error out=w307:errorcluster, "Wire"=w308:refnum<vi>)  [unwired: 1 out]
                      n122 = invoke class="Wire" method="Delete"(reference=w308, error in=w307) -> (error out=w306:errorcluster)  [unwired: 1 in, 2 out]
                    }
                    frame True {
                    }
                  }
                }
                n123 = stacked-sequence {
                  tunnel: w232 -> [w256]
                  tunnel: w231 -> [w250]
                  tunnel: w230 -> [w255]
                  tunnel: [w249] -> w229
                  frame #0 {
                    n124 = Index Array(array=w256, index=w255) -> (element=w254:refnum<vi>)
                    n125 = property class="Term"(reference=w254, error in=w250) -> (error out=w251:errorcluster, "Wire"=w252:refnum<vi>)  [unwired: 1 out]
                    n126 = Not A Number/Path/Refnum?(number/path/refnum=w252) -> (NaN/Path/Refnum?=w253:bool)
                    n127 = case shown="False" w253 {
                      tunnel: w252 -> [w261 _]
                      tunnel: w251 -> [w260 w262]
                      tunnel: [w257 w262] -> w249
                      frame False {
                        n128 = invoke class="Wire" method="RemoveLooseEnds"(reference=w261, error in=w260) -> (reference out=w259:refnum<vi>, error out=w258:errorcluster)  [unwired: 1 in, 1 out]
                        n129 = Close Reference(reference=w259, error in (no error)=w258) -> (error out=w257:errorcluster)
                      }
                      frame True {
                      }
                    }
                  }
                }
                n130 = Close Reference(reference=w232, error in (no error)=w229) -> (error out=w242:errorcluster)
              }
            }
          }
          frame False {
          }
        }
        n131 = Close Reference(reference=w24, error in (no error)=w26) -> (error out=w25:errorcluster)
      }
    }
    frame Error {
    }
  }
  "error out" <- w7
  "ViRefOut" <- "ViRef"
